vi "FRIC_navX_Internal_ProcessingLoop_UpdateAE.vi"(0 "Device Number":T1) -> ()   [LabVIEW 2025]
uses:
  _TypeDefs/Flags/Z900_navX_Flags_HardwareRevTypeDef.ctl
  _TypeDefs/Flags/Z900_navX_Flags_OmnimountConfigTypeDef.ctl
  _TypeDefs/Flags/Z900_navX_Flags_OpStatusTypeDef.ctl
  _TypeDefs/Flags/Z900_navX_Flags_CalibrationStatusTypeDef.ctl
  _TypeDefs/FRIC_navX_DeviceNumbersTypeDef.ctl
panel:
  out "Timestamp":u32
  out "YRPHfH":T2 {"Yaw" format="%.2f"; "Roll" format="%.2f"; "Pitch" format="%.2f"; "Heading" format="%.2f"; "Fused" format="%.2f"}
  out "Status":T5 {"OP Status" items=["INITIALIZING", "SELFTEST_IN_PROGRESS", "ERROR", "IMU_AUTOCAL_IN_PROGRESS", "NORMAL"]; "Calibration Status" items=["IMU_CAL_STATE_MASK"=3, "IMU_CAL_STATE_INPROGRESS"=0, "IMU_CAL_STATE_ACCUMULATE"=1, "IMU_CAL_STATE_COMPLETE"=2]}
  out "Quaternion":T6 {"Quat W" format="%.8f"; "Quat X" format="%.8f"; "Quat Y" format="%.8f"; "Quat Z" format="%.8f"}
  out "Raw Values":T7 {"Accel X" format="%.8f"; "Accel Y" format="%.8f"; "Accel Z" format="%.8f"; "Gyro X" format="%.8f"; "Gyro Y" format="%.8f"; "Gyro Z" format="%.8f"; "Mag X" format="%.8f"; "Mag Y" format="%.8f"; "Mag Z" format="%.8f"}
  out "Linear Acceleration":cluster{"X":dbl, "Y":dbl, "Z":dbl} {"X" format="%_3g"; "Y" format="%_3g"; "Z" format="%_3g"}
  out "Board Information":T10 {"Board"."Hardware Revision" items=["navX-MXP"=33, "navX-Micro"=40]; "Omnimount Config" items=["DEFAULT", "X_UP", "X_DOWN", "Y_UP", "Y_DOWN", "Z_UP", "Z_DOWN"]}
  out "MPUTemp":dbl
  out "Displacement":T11 {"Velocity X" format="%.8f"; "Velocity Y" format="%.8f"; "Velocity Z" format="%.8f"; "Displacement X" format="%.8f"; "Displacement Y" format="%.8f"; "Displacement Z" format="%.8f"}
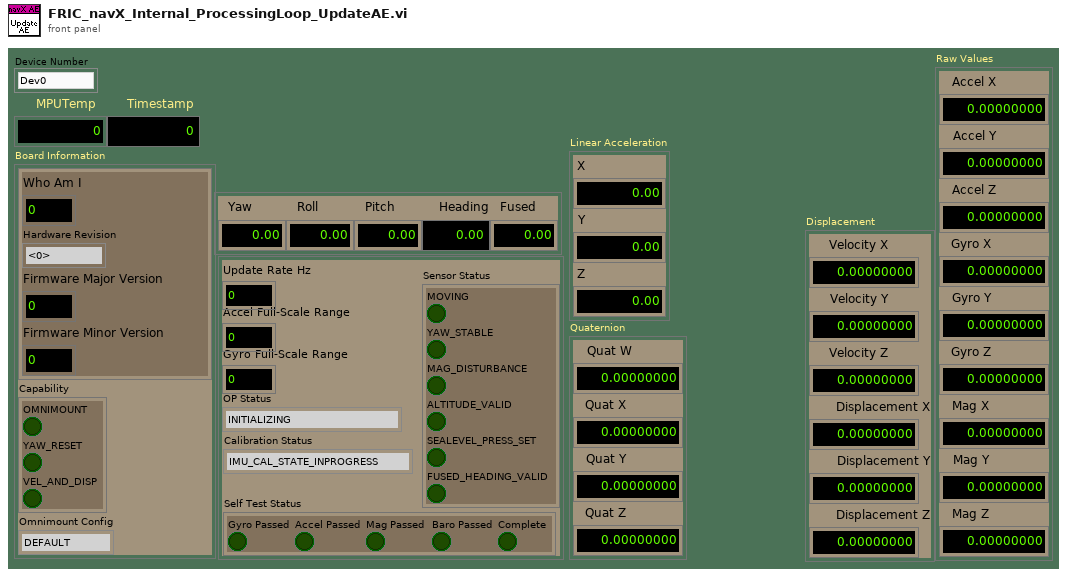
[diagram p1: front panel]
types:
  T1 = typedef "FRIC_navX_DeviceNumbersTypeDef.ctl" = enum16{"Dev0", "Dev1", "Dev2", "Dev3"}
  T2 = cluster{"Yaw":dbl, "Roll":dbl, "Pitch":dbl, "Heading":dbl, "Fused":dbl}
  T3 = typedef "Z900_navX_Flags_OpStatusTypeDef.ctl" = u8
  T4 = typedef "Z900_navX_Flags_CalibrationStatusTypeDef.ctl" = u8
  T5 = cluster{"Update Rate Hz":u8, "Accel Full-Scale Range":u8, "Gyro Full-Scale Range":u16, "OP Status":T3, "Calibration Status":T4, "Sensor Status":cluster{"MOVING":bool, "YAW_STABLE":bool, "MAG_DISTURBANCE":bool, "ALTITUDE_VALID":bool, "SEALEVEL_PRESS_SET":bool, "FUSED_HEADING_VALID":bool}, "Self Test Status":cluster{"Gyro Passed":bool, "Accel Passed":bool, "Mag Passed":bool, "Baro Passed":bool, "Complete":bool}}
  T6 = cluster{"Quat W":dbl, "Quat X":dbl, "Quat Y":dbl, "Quat Z":dbl}
  T7 = cluster{"Accel X":dbl, "Accel Y":dbl, "Accel Z":dbl, "Gyro X":dbl, "Gyro Y":dbl, "Gyro Z":dbl, "Mag X":dbl, "Mag Y":dbl, "Mag Z":dbl}
  T8 = typedef "Z900_navX_Flags_HardwareRevTypeDef.ctl" = u8
  T9 = typedef "Z900_navX_Flags_OmnimountConfigTypeDef.ctl" = u8
  T10 = cluster{"Board":cluster{"Who Am I":u8, "Hardware Revision":T8, "Firmware Major Version":u8, "Firmware Minor Version":u8}, "Capability":cluster{"OMNIMOUNT":bool, "YAW_RESET":bool, "VEL_AND_DISP":bool}, "Omnimount Config":T9}
  T11 = cluster{"Velocity X":dbl, "Velocity Y":dbl, "Velocity Z":dbl, "Displacement X":dbl, "Displacement Y":dbl, "Displacement Z":dbl}
  T12 = cluster{"LinearAcceleration X":dbl, "LinearAcceleration Y":dbl, "LinearAcceleration Z":dbl}
  T13 = cluster{"Update Rate Hz":u8, "Accelerometer Full-Scale Range":u8, "Gyro Full-Scale Range":u16, "OP Status":T3, "Calibration Status":T4, "Sensor Status":cluster{"MOVING":bool, "YAW_STABLE":bool, "MAG_DISTURBANCE":bool, "ALTITUDE_VALID":bool, "SEALEVEL_PRESS_SET":bool, "FUSED_HEADING_VALID":bool}, "Self Test Status":cluster{"Gyro Passed":bool, "Accel Passed":bool, "Mag Passed":bool, "Baro Passed":bool, "Complete":bool}}
  T14 = cluster{"Yaw":dbl, "Roll":dbl, "Pitch":dbl, "Heading":dbl, "Fused Heading":dbl}
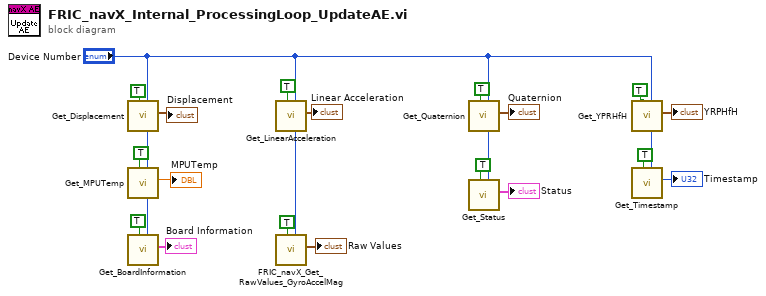
[diagram p0: block diagram]
diagram:
  n1 = call "Get_Displacement.vi"("Device Number"="Device Number", "Update"=TRUE) -> ("Displacement"=→"Displacement":T11)  [unwired: 9 in]
  n2 = call "Get_MPUTemp.vi"("Device Number"="Device Number", "Update"=TRUE) -> ("MPUTemp"=→"MPUTemp":dbl)  [unwired: 9 in]
  n3 = call "Get_BoardInformation.vi"("Device Number"="Device Number", "Update"=TRUE) -> ("Board Information"=→"Board Information":T10)  [unwired: 9 in]
  n4 = call "Get_LinearAcceleration.vi"("Device Number"="Device Number", "Update"=TRUE) -> ("Linear Acceleration"=→"Linear Acceleration":T12)  [unwired: 9 in]
  n5 = call "FRIC_navX_Get_RawValues_GyroAccelMag.vi"("Device Number"="Device Number", "Update"=TRUE) -> ("Raw Values (out)"=→"Raw Values":T7)  [unwired: 9 in]
  n6 = call "Get_Quaternion.vi"("Device Number"="Device Number", "Update"=TRUE) -> ("Quaternion"=→"Quaternion":T6)  [unwired: 9 in]
  n7 = call "Get_Status.vi"("Device Number"="Device Number", "Update"=TRUE) -> ("Status"=→"Status":T13)  [unwired: 9 in]
  n8 = call "Get_YPRHfH.vi"("Device Number"="Device Number", "Update"=TRUE) -> ("YRPHfH"=→"YRPHfH":T14)  [unwired: 9 in]
  n9 = call "Get_Timestamp.vi"("Device Number"="Device Number", "Update"=TRUE) -> ("Timestamp"=→"Timestamp":u32)  [unwired: 9 in]
